vi "Set and Get Active Cell Justify.vi"(7 "Mode":T1, 8 "错误输入":errorcluster, 10 "Justify In":enum16{"Left", "Center", "Right"}(ring), 11 "Mlistbox Ref":refnum<vi>) -> (0 "错误输出":errorcluster, 2 "Justify Out":enum16{"Left", "Center", "Right"}(ring), 3 "Mlistbox Ref Dup":refnum<vi>)   [LabVIEW 2011, in "Mlistbox Tools.lvlib"]
uses:
  Mlistbox Tools.lvlib
  ListBox/Custom Type/Read and Write Mode.ctl
  ListBox/Listbox Tool.lvlib
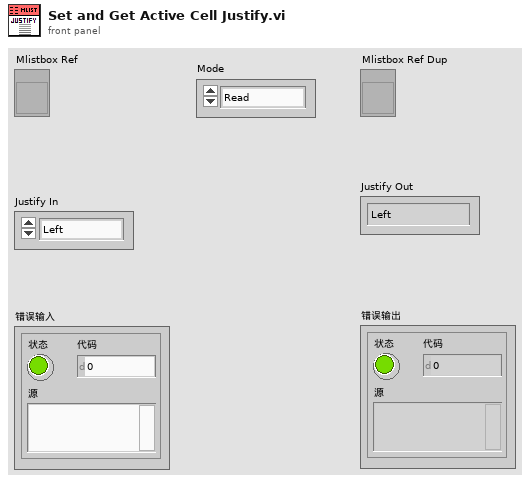
[diagram p1: front panel]
types:
  T1 = typedef "Listbox Tool.lvlib/Read and Write Mode.ctl" = enum16{"Read", "Write"}
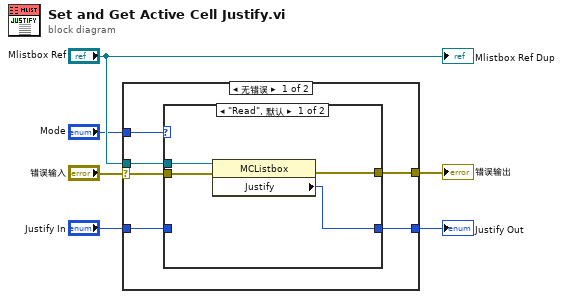
[diagram p0: block diagram]
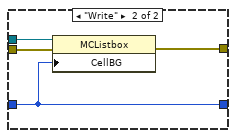
[diagram p2: hidden frame]
diagram:
  n1 = case shown="无错误" "错误输入" {
    selector: "错误输入" -> [w10 w21]
    tunnel: [w8 w21] -> w5
    tunnel: "Mlistbox Ref" -> [w11 _]
    tunnel: "Mode" -> [w12 _]
    tunnel: [w9 _] -> w2
    tunnel: "Justify In" -> [w7 _]
    frame No Error {
      n2 = case shown="\"Read\", 默认" w12 {
        tunnel: w11 -> [w16 w20]
        tunnel: w10 -> [w15 w19]
        tunnel: [w14 w17] -> w9
        tunnel: [w13 w18] -> w8
        tunnel: w7 -> [_ w17]
        frame "Read", Default {
          n3 = property class="MCListbox"(reference=w16, error in=w15) -> (error out=w13:errorcluster, "Justify"=w14:enum16{"Left", "Center", "Right"})  [unwired: 1 out]
        }
        frame "Write" {
          n4 = property class="MCListbox"(reference=w20, error in=w19, "CellBG"=w17) -> (error out=w18:errorcluster)  [unwired: 1 out]
        }
      }
    }
    frame Error {
    }
  }
  "错误输出" <- w5
  "Justify Out" <- w2
  "Mlistbox Ref Dup" <- "Mlistbox Ref"
